vi "CSC_SaveCableConfig.vi"(8 "error in (no error)":errorcluster, 11 "CSC in":refnum<class "CableSerialChain.lvclass">) -> (0 "error out":errorcluster, 3 "CSC out":refnum<class "CableSerialChain.lvclass">)   [LabVIEW 2015, in "CableSerialChain.lvclass"]
uses:
  CableSerialChain.lvclass
  CableSerialChain.lvclass/CableSerialChain.ctl
  <vilib>/Analysis/BLAS.llb/dgemv - General Matrix-Vector Product (DBL).vi
  <vilib>/Analysis/NI_AALBLAS.lvlib
panel:
  out "dgemv":dbl[][](array[numeric])
  out "Coord4":dbl[][](array[numeric])
  out "Array":i32[][](array[numeric])
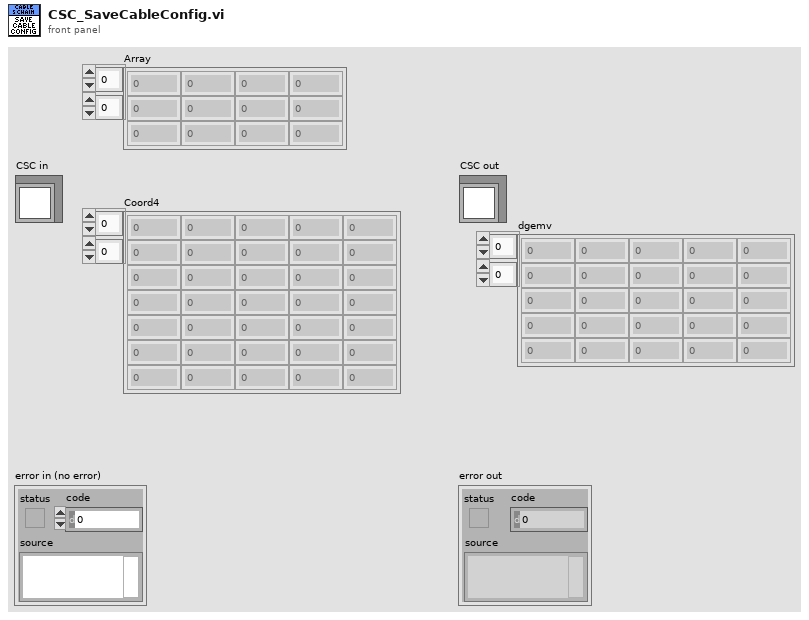
[diagram p1: front panel]
types:
  T1 = typedef "CableSerialChain.lvclass/Cable.ctl" = cluster{"RoutingPtsInLCS":T2[], "Cable ID":i32, "ActiveSegments":i32[][]}
  T2 = typedef "Bodies.lvclass/PointOnBody.ctl" = cluster{"Coord4":dbl[], "ID":i32}
  T3 = typedef "CableSerialChain.lvclass/Cuff.ctl" = cluster{"BodyID":i32, "CoM(CuffCS)":T2, "Mass(kg)":dbl, "CablePts(CuffCS)":T2[], "Cuff->Body":T4}
  T4 = typedef "NI_Matrix.lvlib/RealMatrix.ctl" = dbl[][]
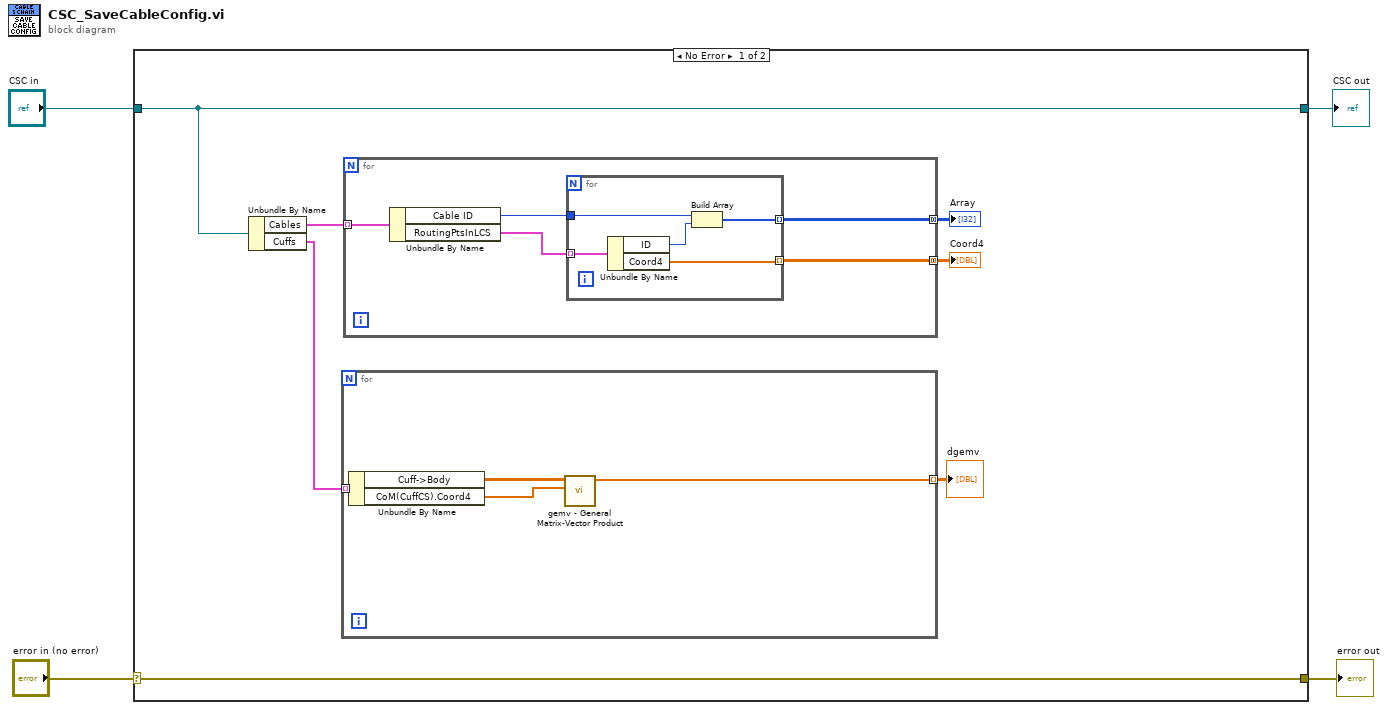
[diagram p0: block diagram]
diagram:
  n1 = case shown="No Error" "error in (no error)" {
    selector: "error in (no error)" -> [w11 w27]
    tunnel: [w11 w27] -> w3
    tunnel: [w10 w26] -> w1
    tunnel: "CSC in" -> [w10 w26]
    frame No Error {
      n2 = Unbundle By Name(w10) -> ("Cables"=w9:T1[], "Cuffs"=w6:T3[])
      n3 = for {
        tunnel: w6 -> [w15] mode=indexing
        tunnel: [w12] -> w5 mode=indexing
        n4 = Unbundle By Name(w15) -> ("Cuff->Body"=w14:T4, "CoM(CuffCS).Coord4"=w13:dbl[])
        n5 = call-poly <vilib>:"gemv - General Matrix-Vector Product.vi"("x"=w13, "A"=w14) -> ("dgemv"=w12:dbl[])  [unwired: 8 in, 1 out]
      }
      "dgemv" <- w5
      n6 = for {
        tunnel: w9 -> [w20] mode=indexing
        tunnel: [w17] -> w8 mode=concatenating
        tunnel: [w16] -> w7 mode=concatenating
        n7 = Unbundle By Name(w20) -> ("Cable ID"=w19:i32, "RoutingPtsInLCS"=w18:T2[])
        n8 = for {
          tunnel: w18 -> [w25] mode=indexing
          tunnel: [w24] -> w16 mode=indexing
          tunnel: w19 -> [w23]
          tunnel: [w21] -> w17 mode=indexing
          n9 = Unbundle By Name(w25) -> ("ID"=w22:i32, "Coord4"=w24:dbl[])
          n10 = Build Array(w23, w22) -> (w21:i32[])
        }
      }
      "Array" <- w8
      "Coord4" <- w7
    }
    frame Error {
    }
  }
  "error out" <- w3
  "CSC out" <- w1
